vi "mDNS Query.vi"(7 "timeout, ms (5000)":i32=5000, 8 "error in (no error)":errorcluster, 10 "max number of responses (all)":u32, 11 "request":T1 {"header"."opcode" items=["Query"=0, "IQuery"=1, "Status"=2, "Notify"=4, "Update"=5, "DSO"=6]; "questions"."class" items=["IN"=1, "CH"=3, "HS"=4, "NONE"=254, "*"=255]; "questions"."type" items=["A"=1, "NS"=2, "MD"=3, "MF"=4, "CNAME"=5, "SOA"=6, "MB"=7, "MG"=8, "MR"=9, "NULL"=10, "WKS"=11, "PTR"=12, "HINFO"=13, "MINFO"=14, "MX"=15, "TXT"=16, "RP"=17, "AFSDB"=18, "X25"=19, "ISDN"=20, "RT"=21, "NSAP"=22, "NSAP-PTR"=23, "SIG"=24, "KEY"=25, "PX"=26, "GPOS"=27, "AAAA"=28, "LOC"=29, "NXT"=30, "EID"=31, "NIMLOC"=32, "SRV"=33, "ATMA"=34, "NAPTR"=35, "KX"=36, "CERT"=37, "A6"=38, "DNAME"=39, "SINK"=40, "OPT"=41, "APL"=42, "DS"=43, "SSHFP"=44, "IPSECKEY"=45, "RRSIG"=46, "NSEC"=47, "DNSKEY"=48, "DHCID"=49, "NSEC3"=50, "NSEC3PARAM"=51, "TLSA"=52, "SMIMEA"=53, "HIP"=55, "NINFO"=56, "RKEY"=57, "TALINK"=58, "CDS"=59, "CDNSKEY"=60, "OPENPGPKEY"=61, "CSYNC"=62, "ZONEMD"=63, "SVCB"=64, "HTTPS"=65, "SPF"=99, "UINFO"=100, "UID"=101, "GID"=102, "UNSPEC"=103, "NID"=104, "L32"=105, "L64"=106, "LP"=107, "EUI48"=108, "EUI64"=109, "TKEY"=249, "TSIG"=250, "IXFR"=251, "AXFR"=252, "MAILB"=253, "MAILA"=254, "*"=255, "URI"=256, "CAA"=257, "AVC"=258, "DOA"=259, "AMTRELAY"=260, "TA"=32768, "DLV"=32769]}) -> (0 "error out":errorcluster, 3 "responses":T2(array[cluster]) {"header"."response code" items=["NoError"=0, "FormErr"=1, "ServFail"=2, "NXDomain"=3, "NotImp"=4, "Refused"=5, "YXDomain"=6, "YXRRSet"=7, "NXRRSet"=8, "NotAuth"=9, "NotZone"=10, "DSOTYPENI"=11, "BADVERS/BADSIG"=16, "BADKEY"=17, "BADTIME"=18, "BADMODE"=19, "BADNAME"=20, "BADALG"=21, "BADTRUNC"=22, "BADCOOKIE"=23]; "header"."opcode" items=["Query"=0, "IQuery"=1, "Status"=2, "Notify"=4, "Update"=5, "DSO"=6]; "additional records"."class" items=["IN"=1, "CH"=3, "HS"=4]; "additional records"."type" items=["A"=1, "NS"=2, "MD"=3, "MF"=4, "CNAME"=5, "SOA"=6, "MB"=7, "MG"=8, "MR"=9, "NULL"=10, "WKS"=11, "PTR"=12, "HINFO"=13, "MINFO"=14, "MX"=15, "TXT"=16, "RP"=17, "AFSDB"=18, "X25"=19, "ISDN"=20, "RT"=21, "NSAP"=22, "NSAP-PTR"=23, "SIG"=24, "KEY"=25, "PX"=26, "GPOS"=27, "AAAA"=28, "LOC"=29, "NXT"=30, "EID"=31, "NIMLOC"=32, "SRV"=33, "ATMA"=34, "NAPTR"=35, "KX"=36, "CERT"=37, "A6"=38, "DNAME"=39, "SINK"=40, "OPT"=41, "APL"=42, "DS"=43, "SSHFP"=44, "IPSECKEY"=45, "RRSIG"=46, "NSEC"=47, "DNSKEY"=48, "DHCID"=49, "NSEC3"=50, "NSEC3PARAM"=51, "TLSA"=52, "SMIMEA"=53, "HIP"=55, "NINFO"=56, "RKEY"=57, "TALINK"=58, "CDS"=59, "CDNSKEY"=60, "OPENPGPKEY"=61, "CSYNC"=62, "ZONEMD"=63, "SVCB"=64, "HTTPS"=65, "SPF"=99, "UINFO"=100, "UID"=101, "GID"=102, "UNSPEC"=103, "NID"=104, "L32"=105, "L64"=106, "LP"=107, "EUI48"=108, "EUI64"=109, "URI"=256, "CAA"=257, "AVC"=258, "DOA"=259, "AMTRELAY"=260, "TA"=32768, "DLV"=32769]; "authority records"."class" items=["IN"=1, "CH"=3, "HS"=4]; "authority records"."type" items=["A"=1, "NS"=2, "MD"=3, "MF"=4, "CNAME"=5, "SOA"=6, "MB"=7, "MG"=8, "MR"=9, "NULL"=10, "WKS"=11, "PTR"=12, "HINFO"=13, "MINFO"=14, "MX"=15, "TXT"=16, "RP"=17, "AFSDB"=18, "X25"=19, "ISDN"=20, "RT"=21, "NSAP"=22, "NSAP-PTR"=23, "SIG"=24, "KEY"=25, "PX"=26, "GPOS"=27, "AAAA"=28, "LOC"=29, "NXT"=30, "EID"=31, "NIMLOC"=32, "SRV"=33, "ATMA"=34, "NAPTR"=35, "KX"=36, "CERT"=37, "A6"=38, "DNAME"=39, "SINK"=40, "OPT"=41, "APL"=42, "DS"=43, "SSHFP"=44, "IPSECKEY"=45, "RRSIG"=46, "NSEC"=47, "DNSKEY"=48, "DHCID"=49, "NSEC3"=50, "NSEC3PARAM"=51, "TLSA"=52, "SMIMEA"=53, "HIP"=55, "NINFO"=56, "RKEY"=57, "TALINK"=58, "CDS"=59, "CDNSKEY"=60, "OPENPGPKEY"=61, "CSYNC"=62, "ZONEMD"=63, "SVCB"=64, "HTTPS"=65, "SPF"=99, "UINFO"=100, "UID"=101, "GID"=102, "UNSPEC"=103, "NID"=104, "L32"=105, "L64"=106, "LP"=107, "EUI48"=108, "EUI64"=109, "URI"=256, "CAA"=257, "AVC"=258, "DOA"=259, "AMTRELAY"=260, "TA"=32768, "DLV"=32769]; "answers"."class" items=["IN"=1, "CH"=3, "HS"=4]; "answers"."type" items=["A"=1, "NS"=2, "MD"=3, "MF"=4, "CNAME"=5, "SOA"=6, "MB"=7, "MG"=8, "MR"=9, "NULL"=10, "WKS"=11, "PTR"=12, "HINFO"=13, "MINFO"=14, "MX"=15, "TXT"=16, "RP"=17, "AFSDB"=18, "X25"=19, "ISDN"=20, "RT"=21, "NSAP"=22, "NSAP-PTR"=23, "SIG"=24, "KEY"=25, "PX"=26, "GPOS"=27, "AAAA"=28, "LOC"=29, "NXT"=30, "EID"=31, "NIMLOC"=32, "SRV"=33, "ATMA"=34, "NAPTR"=35, "KX"=36, "CERT"=37, "A6"=38, "DNAME"=39, "SINK"=40, "OPT"=41, "APL"=42, "DS"=43, "SSHFP"=44, "IPSECKEY"=45, "RRSIG"=46, "NSEC"=47, "DNSKEY"=48, "DHCID"=49, "NSEC3"=50, "NSEC3PARAM"=51, "TLSA"=52, "SMIMEA"=53, "HIP"=55, "NINFO"=56, "RKEY"=57, "TALINK"=58, "CDS"=59, "CDNSKEY"=60, "OPENPGPKEY"=61, "CSYNC"=62, "ZONEMD"=63, "SVCB"=64, "HTTPS"=65, "SPF"=99, "UINFO"=100, "UID"=101, "GID"=102, "UNSPEC"=103, "NID"=104, "L32"=105, "L64"=106, "LP"=107, "EUI48"=108, "EUI64"=109, "URI"=256, "CAA"=257, "AVC"=258, "DOA"=259, "AMTRELAY"=260, "TA"=32768, "DLV"=32769]})   [LabVIEW 2015, in "PL DNS Client.lvlib"]
doc: "Sends Multicast DNS query and parses received responses. <b>max number of responses</b> can be used to limit the number of responses to receive."
uses:
  PL DNS Client.lvlib
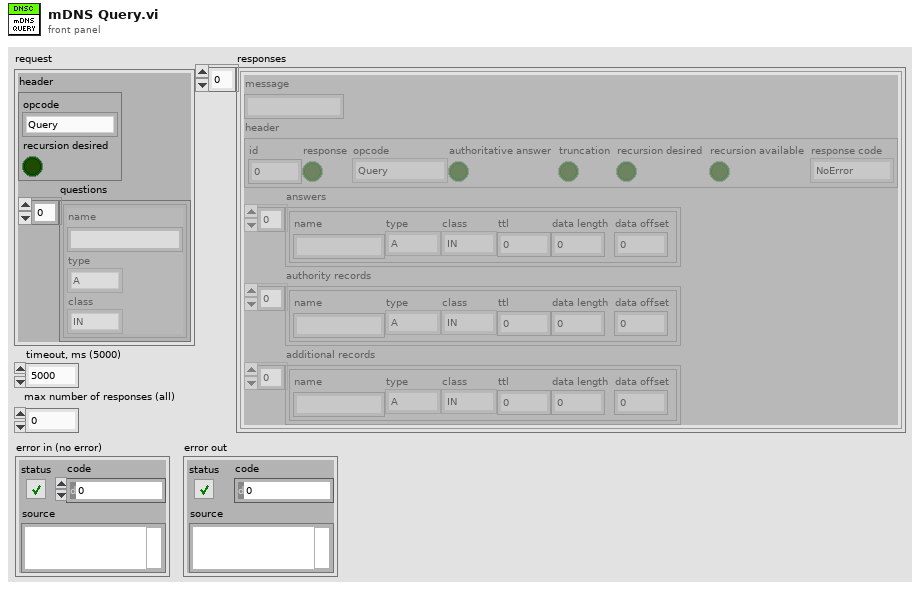
[diagram p1: front panel]
types:
  T1 = cluster{"header":cluster{"opcode":u8, "recursion desired":bool}, "questions":cluster{"name":string, "type":u16, "class":u16}[]}
  T2 = cluster{"message":string, "header":cluster{"id":u16, "response":bool, "opcode":u8, "authoritative answer":bool, "truncation":bool, "recursion desired":bool, "recursion available":bool, "response code":u16}, "answers":cluster{"name":string, "type":u16, "class":u16, "ttl":u32, "data length":u16, "data offset":u16}[], "authority records":cluster{"name":string, "type":u16, "class":u16, "ttl":u32, "data length":u16, "data offset":u16}[], "additional records":cluster{"name":string, "type":u16, "class":u16, "ttl":u32, "data length":u16, "data offset":u16}[]}[]
  T3 = cluster{"message":string, "header":cluster{"id":u16, "response":bool, "opcode":u8, "authoritative answer":bool, "truncation":bool, "recursion desired":bool, "recursion available":bool, "response code":u16}, "answers":cluster{"name":string, "type":u16, "class":u16, "ttl":u32, "data length":u16, "data offset":u16}[], "authority records":cluster{"name":string, "type":u16, "class":u16, "ttl":u32, "data length":u16, "data offset":u16}[], "additional records":cluster{"name":string, "type":u16, "class":u16, "ttl":u32, "data length":u16, "data offset":u16}[]}
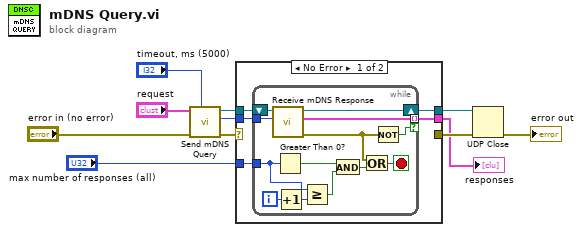
[diagram p0: block diagram]
diagram:
  n1 = call "Send mDNS Query.vi"("timeout, ms (5000)"="timeout, ms (5000)", "error in (no error)"="error in (no error)", "query"="request") -> ("error out"=w8:errorcluster, "query id"=w2:u16, "connection ID"=w7:refnum<k16>)  [unwired: 6 in]
  n2 = case shown="No Error" w8 {
    selector: w8 -> [_ w30]
    tunnel: w7 -> [w16 w31]
    tunnel: [w15 w31] -> w6
    tunnel: [_ w30] -> w5
    tunnel: [w14 _] -> w3
    tunnel: w2 -> [w13 _]
    tunnel: "max number of responses (all)" -> [w12 _]
    frame No Error {
      n3 = while {
        shift-right: [w28] -> w15
        shift-left: w16 -> [w29]
        tunnel: [w27] -> w14 mode=indexing if=w26
        tunnel: w13 -> [w25]
        tunnel: w12 -> [w19]
        i -> [w21]
        stop <- w24 stop-if-true
        n4 = call "Receive mDNS Response.vi"("query id"=w25, "connection ID"=w29) -> ("error out"=w23:errorcluster, "response"=w27:T3, "connection ID out"=w28:refnum<k16>)  [unwired: 7 in]
        n5 = Greater Than 0?(x=w19) -> (x > 0?=w22:bool)
        n6 = Increment(x=w21) -> (x+1=w20:i32)
        n7 = Greater Or Equal?(x=w19, y=w20) -> (x >= y?=w18:bool)
        n8 = And(x=w22, y=w18) -> (x .and. y?=w17:bool)
        n9 = Or(x=w23, y=w17) -> (x .or. y?=w24:bool)
        n10 = Not(x=w23) -> (.not. x?=w26:bool)
      }
    }
    frame Error {
    }
  }
  "responses" <- w3
  n11 = UDP Close(connection ID=w6, 8:w5) -> (error out=→"error out":errorcluster)  [unwired: 1 out]
